vi "SetVCLKReg_SD.vi"(0 "vfreq":u8, 1 "lines":u32) -> ()   [LabVIEW 2015]
uses:
  DLL/ESLSCDLL.dll
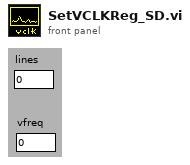
[diagram p1: front panel]
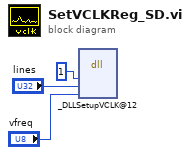
[diagram p0: block diagram]
diagram:
  n1 = dll-call lib="G:/SD/TRANCON-2015/DLL/ESLSCDLL.dll" fn="_DLLSetupVCLK@12" ("lwlscdll.dll:DLLSetupVCLK")("drv"=u32 1, "lines"="lines", "vfreq"="vfreq") -> ()  [unwired: 7 in, 2 out]
